vi "LittleEndianToInt16.vi"(11 "Little endian int string":string) -> (3 "Int16 value":i16)   [LabVIEW 2020]
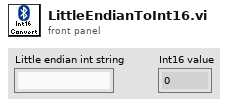
[diagram p1: front panel]
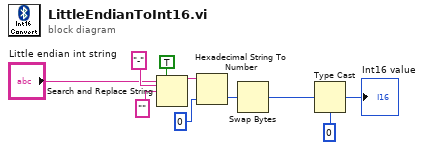
[diagram p0: block diagram]
diagram:
  n1 = Search and Replace String(replace all?=TRUE ("replace all? (F)"), input string="Little endian int string", search string="-", replace string="" ("replace string (\"\")")) -> (result string=w7:string)  [unwired: 4 in, 3 out]
  n2 = Hexadecimal String To Number(string=w7, default (0uL)=i16 0 ("default (0 U32)")) -> (number=w6:i16)  [unwired: 1 in, 1 out]
  n3 = Swap Bytes(anything=w6) -> (byte swapped=w3:i16)
  n4 = Type Cast(type=i16 0, x=w3) -> (*(type *) &x=→"Int16 value":i16)
